vi "File path.vi"(8 "error in (no error)":errorcluster, 10 "Path":path, 11 "Generador de Funciones in":refnum<class "Generador de Funciones.lvclass">) -> (0 "error out":errorcluster, 3 "Generador de Funciones out":refnum<class "Generador de Funciones.lvclass">)   [LabVIEW 2020, in "Generador de Funciones.lvlib" / "Generador de Funciones.lvclass"]
uses:
  Generador de Funciones.lvclass
  Generador de Funciones.lvclass/Generador de Funciones.ctl
  Logging Txt/Logging Txt Messages/Write Path Msg/Write Path Msg.lvclass/Write Path Msg.ctl
  <vilib>/ActorFramework/Message Enqueuer/Message Enqueuer.lvclass/Message Enqueuer.ctl
  <vilib>/ActorFramework/Message Enqueuer/Enqueue.vi
  Logging Txt/Logging Txt Messages/Write Path Msg/Write Path Msg.lvclass
  C:/Program Files (x86)/National Instruments/LabVIEW 2020/vi.lib/ActorFramework/Message/Message.lvclass
  <vilib>/ActorFramework/Message Priority Queue/Priority Enqueue.vi
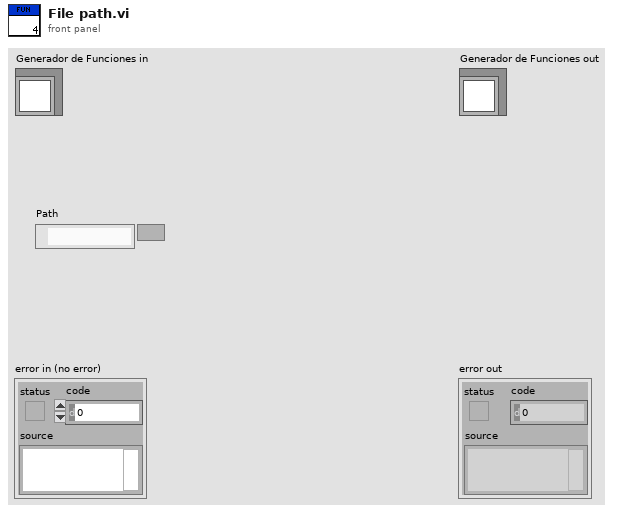
[diagram p1: front panel]
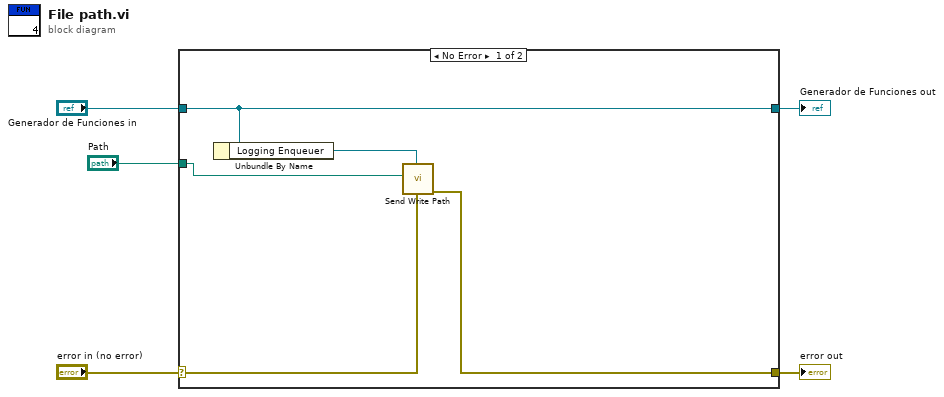
[diagram p0: block diagram]
diagram:
  n1 = case shown="No Error" "error in (no error)" {
    selector: "error in (no error)" -> [w7 w12]
    tunnel: [w6 w12] -> w4
    tunnel: [w10 w11] -> w2
    tunnel: "Generador de Funciones in" -> [w10 w11]
    tunnel: "Path" -> [w8 _]
    frame No Error {
      n2 = Unbundle By Name(w10) -> ("Logging Enqueuer"=w9:refnum<class "Message Enqueuer.lvclass">)
      n3 = call "Send Write Path.vi"("error in (no error)"=w7, "Path"=w8, "Message Enqueuer"=w9) -> ("error out"=w6:errorcluster)  [unwired: 7 in, 1 out]
    }
    frame Error {
    }
  }
  "error out" <- w4
  "Generador de Funciones out" <- w2
